vi "Compile APU 1.0 Data.vi"(8 "error in (no error)":errorcluster, 11 "Device Item Ref in":T3 format="%.0x") -> (0 "error out":errorcluster, 2 "APUs":T1[](array[typedef]) {"shared settings"."cycle start" format="%#.15g"}, 3 "Device Item Ref out":T3 format="%.0x")   [LabVIEW 2015, in "Engine Simulation Toolkit System Explorer.lvlib"]
uses:
  Engine Simulation Toolkit System Explorer.lvlib
  <vilib>/NI Veristand/Custom Device API/Custom Device Item Ref.ctl
  Shared/1.0 APU Engine Data.ctl
  Shared/1.0 APU Engine FIFO Idxs.ctl
  DBL Angle to U16.vi
  Shared/Properties.vi
  Shared/Constants and GUIDs.vi
  <vilib>/NI Veristand/Custom Device Tools/Custom Device Utility Library/NI VeriStand - Search for All Items by GUID.vi
  <vilib>/NI Veristand/Custom Device API/Get Item Property (String).vi
  <vilib>/NI Veristand/Custom Device API/Get Item Property (Double).vi
  <vilib>/NI Veristand/Custom Device API/Get Item Property (Boolean).vi
  <vilib>/NI Veristand/Custom Device API/Get Item Property (U16).vi
  <vilib>/NI Veristand/Custom Device Tools/Custom Device Utility Library/NI VeriStand - Search for Item by GUID.vi
  Shared/Engine Simulation Toolkit Shared.lvlib
  <vilib>/NI Veristand/Custom Device API/Custom Device API.lvlib
  <vilib>/NI Veristand/Custom Device Tools/Custom Device Utility Library/Custom Device Utility Library.lvlib
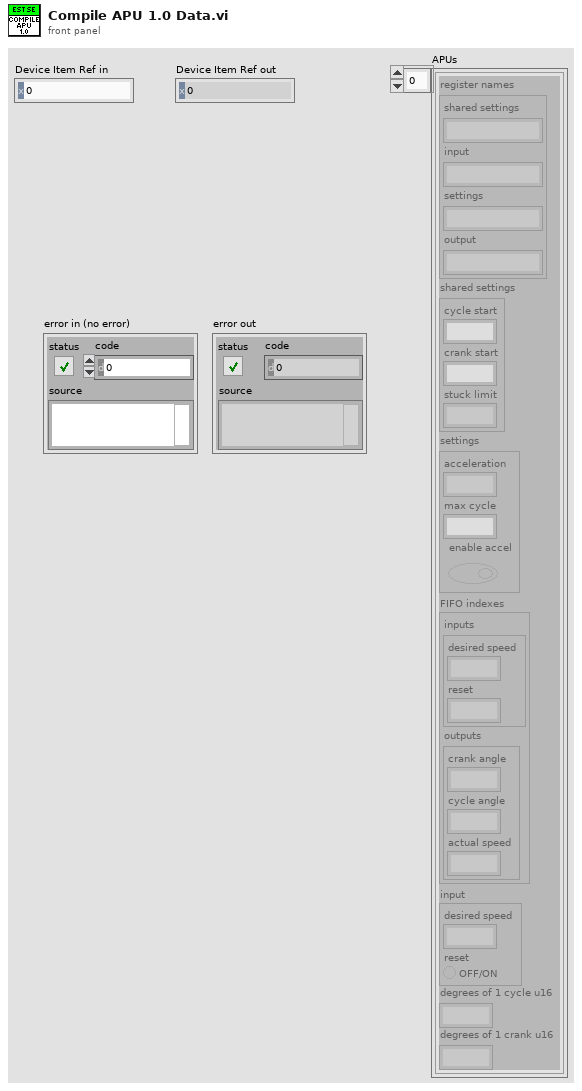
[diagram p1: front panel]
types:
  T1 = typedef "Engine Simulation Toolkit Shared.lvlib/1.0 APU Engine Data.ctl" = cluster{"register names":cluster{"shared settings":string, "input":string, "settings":string, "output":string}, "shared settings":cluster{"cycle start":fxp<+,2,2>, "crank start":u16, "stuck limit":fxp<+,18,18>}, "settings":cluster{"acceleration":fxp<+,18,-20>, "max cycle":fxp<+,2,2>, "enable accel":bool}, "FIFO indexes":T2, "input":cluster{"desired speed":fxp<+/-,23,2>, "reset":bool}, "degrees of 1 cycle u16":dbl, "degrees of 1 crank u16":dbl}
  T2 = typedef "Engine Simulation Toolkit Shared.lvlib/1.0 APU Engine FIFO Idxs.ctl" = cluster{"inputs":cluster{"desired speed":i32, "reset":i32}, "outputs":cluster{"crank angle":i32, "cycle angle":i32, "actual speed":i32}}
  T3 = typedef "Custom Device API.lvlib/Custom Device Item Ref.ctl" = u64
  T4 = typedef "Engine Simulation Toolkit Shared.lvlib/Channel.ctl" = cluster{"Name":string, "Units":string, "Default":dbl, "Description":string}
  T5 = cluster{"desired speed":fxp<+/-,23,2>, "reset":bool}
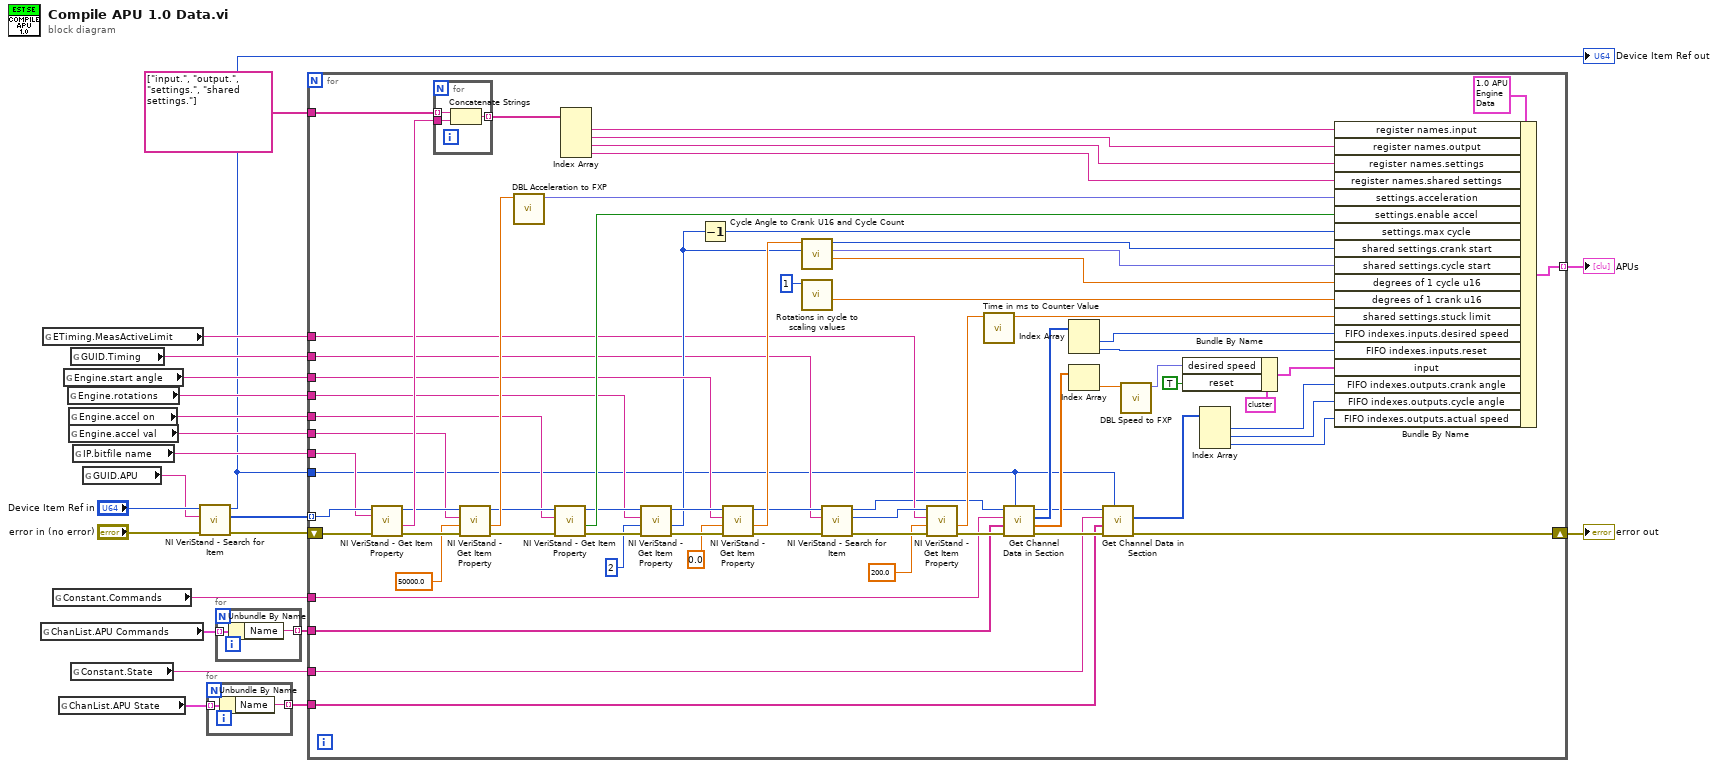
[diagram p0: block diagram]
diagram:
  n1 = global read "Constants and GUIDs.vi" "ChanList.APU Commands"() -> (w5:T4[])
  n2 = global read "Properties.vi" "ETiming.MeasActiveLimit"() -> (w10:string)
  n3 = global read "Constants and GUIDs.vi" "Constant.Commands"() -> (w9:string)
  n4 = global read "Constants and GUIDs.vi" "ChanList.APU State"() -> (w3:T4[])
  n5 = global read "Properties.vi" "Engine.start angle"() -> (w12:string)
  n6 = global read "Properties.vi" "Engine.rotations"() -> (w13:string)
  n7 = global read "Properties.vi" "Engine.accel on"() -> (w14:string)
  n8 = global read "Properties.vi" "Engine.accel val"() -> (w16:string)
  n9 = global read "Constants and GUIDs.vi" "GUID.Timing"() -> (w11:string)
  n10 = global read "Constants and GUIDs.vi" "Constant.State"() -> (w6:string)
  n11 = global read "Properties.vi" "IP.bitfile name"() -> (w18:string)
  n12 = global read "Constants and GUIDs.vi" "GUID.APU"() -> (w20:string)
  n13 = call-poly <vilib>:"NI VeriStand - Search for Item.vi"("error in"="error in (no error)", "Item GUID"=w20, "Section Ref in"="Device Item Ref in") -> ("error out"=w19:errorcluster, "Item Refs"=w1:T3[], "Section Ref out"=w7:T3)  [unwired: 5 in, 1 out]
  "Device Item Ref out" <- w7
  n14 = for {
    tunnel: w3 -> [w24] mode=indexing
    tunnel: [w23] -> w2 mode=indexing
    n15 = Unbundle By Name(w24) -> ("Name"=w23:string)
  }
  n16 = for {
    tunnel: w5 -> [w26] mode=indexing
    tunnel: [w25] -> w4 mode=indexing
    n17 = Unbundle By Name(w26) -> ("Name"=w25:string)
  }
  n18 = for {
    shift-right: [w41] -> w15
    shift-left: w19 -> [w96]
    tunnel: w1 -> [w95] mode=indexing
    tunnel: w18 -> [w94]
    tunnel: string[] ["input.", "output.", "settings.", "shared settings."] -> [w92]
    tunnel: w16 -> [w83]
    tunnel: w14 -> [w77]
    tunnel: w13 -> [w73]
    tunnel: w12 -> [w69]
    tunnel: w11 -> [w60]
    tunnel: w10 -> [w57]
    tunnel: w9 -> [w52]
    tunnel: w4 -> [w28]
    tunnel: [w46] -> w8 mode=indexing
    tunnel: w7 -> [w40]
    tunnel: w6 -> [w38]
    tunnel: w2 -> [w27]
    n19 = call-poly <vilib>:"NI VeriStand - Get Item Property.vi"("error in (no error)"=w96, "Property Name"=w94, "Item Ref in"=w95) -> ("error out"=w84:errorcluster, "Value"=w93:string, "Item Ref out"=w85:T3)  [unwired: 5 in, 1 out]
    n20 = for {
      tunnel: w93 -> [w99]
      tunnel: w92 -> [w98] mode=indexing
      tunnel: [w97] -> w90 mode=indexing
      n21 = Concatenate Strings(w98, w99) -> (w97:string)
    }
    n22 = call-poly <vilib>:"NI VeriStand - Get Item Property.vi"("error in (no error)"=w84, "Default Value"=50000.0, "Property Name"=w83, "Item Ref in"=w85) -> ("error out"=w82:errorcluster, "Value"=w81:dbl, "Item Ref out"=w78:T3)  [unwired: 4 in, 1 out]
    n23 = call "DBL Acceleration to FXP.vi"("Desired acceleration (RPM/sec)"=w81) -> ("FXP acceleration"=w80:fxp<+,18,-20>)  [unwired: 6 in, 4 out]
    n24 = call-poly <vilib>:"NI VeriStand - Get Item Property.vi"("error in (no error)"=w82, "Property Name"=w77, "Item Ref in"=w78) -> ("error out"=w79:errorcluster, "Value"=w76:bool, "Item Ref out"=w74:T3)  [unwired: 5 in, 1 out]
    n25 = Index Array(array=w90) -> (element #1=w89:string, element #2=w88:string, element #3=w87:string, element #4=w86:string)  [unwired: 4 in]
    n26 = call-poly <vilib>:"NI VeriStand - Get Item Property.vi"("error in (no error)"=w79, "Default Value"=u16 2, "Property Name"=w73, "Item Ref in"=w74) -> ("error out"=w75:errorcluster, "Value"=w65:u16, "Item Ref out"=w70:T3)  [unwired: 4 in, 1 out]
    n27 = Decrement(x=w65) -> (x-1=w32:u16)
    n28 = call-poly <vilib>:"NI VeriStand - Get Item Property.vi"("error in (no error)"=w75, "Default Value"=0.0, "Property Name"=w69, "Item Ref in"=w70) -> ("error out"=w71:errorcluster, "Value"=w66:dbl, "Item Ref out"=w61:T3)  [unwired: 4 in, 1 out]
    n29 = call "Cycle Angle to Crank U16 and Cycle Count.vi"("rotations"=w65, "cycle angle"=w66) -> ("degrees of one u16"=w31:dbl, "cycle count"=w63:fxp<+,2,2>, "crank U16"=w64:u16)  [unwired: 7 in]
    n30 = call "Rotations in cycle to scaling values.vi"("rotations in a cycle"=u16 1) -> ("degrees of one u16"=w29:dbl)  [unwired: 8 in, 2 out]
    n31 = call-poly <vilib>:"NI VeriStand - Search for Item.vi"("error in"=w71, "Item GUID"=w60, "Section Ref in"=w61) -> ("error out"=w62:errorcluster, "Item Ref"=w58:T3, "Section Ref out"=w53:T3)  [unwired: 5 in, 1 out]
    n32 = call-poly <vilib>:"NI VeriStand - Get Item Property.vi"("error in (no error)"=w62, "Default Value"=200.0, "Property Name"=w57, "Item Ref in"=w58) -> ("error out"=w59:errorcluster, "Value"=w55:dbl)  [unwired: 4 in, 2 out]
    n33 = call "Time in ms to Counter Value.vi"("time (ms)"=w55) -> ("counter value"=w54:dbl)  [unwired: 10 in]
    n34 = call "Get Channel Data in Section.vi"("Custom device ref"=w40, "error in (no error)"=w59, "Channels"=w28, "Section (\"\":none)"=w52, "Item Ref in"=w53) -> ("error out"=w51:errorcluster, "default values"=w45:dbl[], "FIFO indexes"=w50:i32[], "Item Ref out"=w39:T3)  [unwired: 2 in, 1 out]
    n35 = Index Array(array=w50) -> (element #1=w49:i32, element #2=w48:i32)  [unwired: 2 in]
    n36 = Index Array(array=w45) -> (element=w44:dbl)  [unwired: 1 in]
    n37 = call "Get Channel Data in Section.vi"("Custom device ref"=w40, "error in (no error)"=w51, "Channels"=w27, "Section (\"\":none)"=w38, "Item Ref in"=w39) -> ("error out"=w41:errorcluster, "FIFO indexes"=w37:i32[])  [unwired: 2 in, 3 out]
    n38 = call "DBL Speed to FXP.vi"("Desired speed (RPM)"=w44) -> ("FXP speed"=w42:fxp<+/-,23,2>)  [unwired: 6 in, 4 out]
    n39 = Bundle By Name(cluster=T5 {"desired speed"=0.0, "reset"=FALSE} ("input"), "desired speed"=w42, "reset"=TRUE) -> (w43:T5)
    n40 = Index Array(array=w37) -> (element #1=w36:i32, element #2=w35:i32, element #3=w34:i32)  [unwired: 3 in]
    n41 = Bundle By Name(cluster=T1 {"register names"={"shared settings"="", "input"="", "settings"="", "output"=""}, "shared settings"={"cycle start"=0.0, "crank start"=0, "stuck limit"=0.0}, "settings"={"acceleration"=0.0, "max cycle"=0.0, "enable accel"=FALSE}, "FIFO indexes"={"inputs"={"desired speed"=0, "reset"=0}, "outputs"={"crank angle"=0, "cycle angle"=0, "actual speed"=0}}, "input"={"desired speed"=0.0, "reset"=FALSE}, "degrees of 1 cycle u16"=0.0, "degrees of 1 crank u16"=0.0} ("1.0.0 APU"), "register names.input"=w89, "register names.output"=w88, "register names.settings"=w87, "register names.shared settings"=w86, "settings.acceleration"=w80, "settings.enable accel"=w76, "settings.max cycle"=w32, "shared settings.crank start"=w64, "shared settings.cycle start"=w63, "degrees of 1 cycle u16"=w31, "degrees of 1 crank u16"=w29, "shared settings.stuck limit"=w54, "FIFO indexes.inputs.desired speed"=w49, "FIFO indexes.inputs.reset"=w48, "input"=w43, "FIFO indexes.outputs.crank angle"=w36, "FIFO indexes.outputs.cycle angle"=w35, "FIFO indexes.outputs.actual speed"=w34) -> (w46:T1)
  }
  "error out" <- w15
  "APUs" <- w8
